vi "PWM_Lenkung.vi"(0 "vorne rechts":dbl, 1 "vorne links":dbl, 2 "Schräg rechts":dbl, 4 "Schräg links":dbl, 5 "PID gains out 2":T1={"proportional gain (Kc)"=0.5, "integral time (Ti, min)"=1.0, "derivative time (Td, min)"=0.001} {"proportional gain (Kc)" format="%#_10g"; "integral time (Ti, min)" format="%#_10g"; "derivative time (Td, min)" format="%#_10g"}) -> (14 "PWM Lenkung":dbl)   [LabVIEW 2016]
doc: "PID Regelung für Servowert\n05.04.17_Tloe"
uses:
  <vilib>/addons/control/pid/pid.llb/PID Advanced (DBL).vi
  <vilib>/addons/control/pid/NI_PID_pid.lvlib
panel:
  in  "y":dbl=0.1
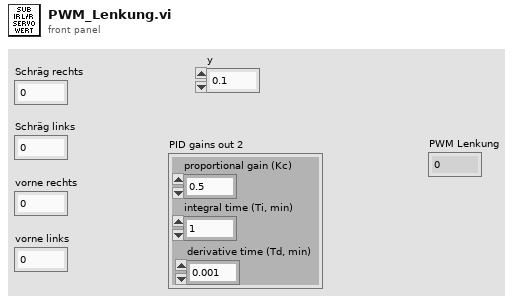
[diagram p1: front panel]
types:
  T1 = cluster{"proportional gain (Kc)":dbl, "integral time (Ti, min)":dbl, "derivative time (Td, min)":dbl}
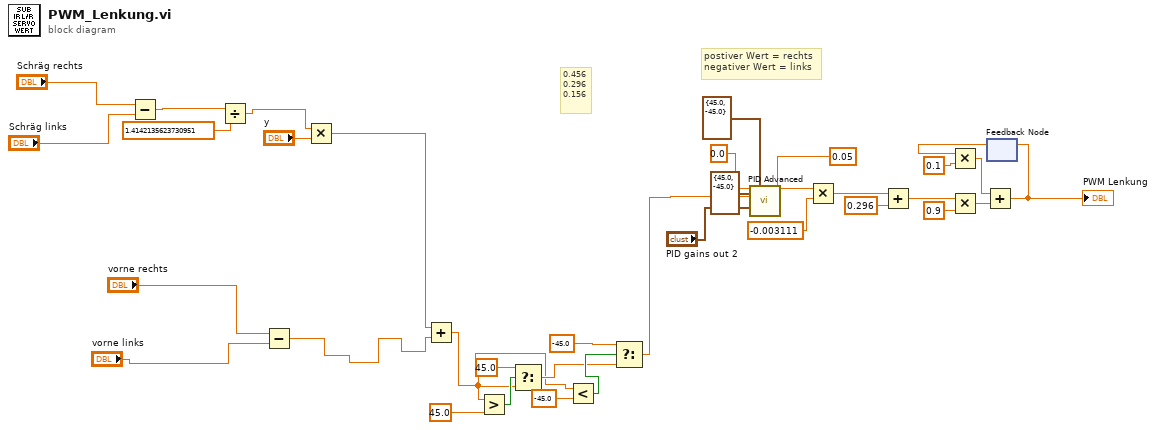
[diagram p0: block diagram]
diagram:
  # "0.456\n0.296\n0.156"
  # "postiver Wert = rechts\nnegativer Wert = links"
  n1 = Subtract(x="Schräg rechts", y="Schräg links") -> (x-y=w17:dbl)
  n2 = Divide(x=w17, y=1.4142135623730951) -> (x/y=w15:dbl)
  n3 = Subtract(x="vorne rechts", y="vorne links") -> (x-y=w1:dbl)
  n4 = Multiply(x=w15, y="y") -> (x*y=w4:dbl)
  n5 = Add(x=w4, y=w1) -> (x+y=w3:dbl)
  n6 = Greater?(x=w3, y=45.0) -> (0:w13:bool)
  n7 = Select(t=45.0, s=w13, f=w3) -> (s? t:f=w7:dbl)
  n8 = Less?(x=w3, y=-45.0) -> (x < y?=w8:bool)
  n9 = Select(t=-45.0, s=w8, f=w7) -> (s? t:f=w6:dbl)
  n10 = call-poly <vilib>:"PID Advanced.vi"("setpoint"=0.0, "output range"=cluster{"output high":dbl, "output low":dbl} {"output high"=45.0, "output low"=-45.0}, "process variable"=w6, "setpoint range"=cluster{"setpoint high":dbl, "setpoint low":dbl} {"setpoint high"=45.0, "setpoint low"=-45.0}, "alpha"=0.05, "PID gains"="PID gains out 2") -> ("output"=w35:dbl)  [unwired: 8 in, 1 out]
  n11 = Multiply(x=w35, y=-0.003111) -> (x*y=w31:dbl)
  n12 = Add(x=w31, y=0.296) -> (x+y=w33:dbl)
  n13 = Multiply(x=w33, y=0.9) -> (x*y=w29:dbl)
  n14 = feedback #1() -> (w24:dbl)  [unwired: 1 in]
  n15 = Multiply(x=w24, y=0.1) -> (x*y=w28:dbl)
  n16 = Add(x=w28, y=w29) -> (x+y=w25:dbl)
  "PWM Lenkung" <- w25
  n17 = feedback-in #1(w25) -> ()
